vi "Make DLL Param(Read Storage Rsp).vi"(1 "Read Storage Rsp":T2) -> (0 "pRsp":T1)   [LabVIEW 8.6, in "Keyence LJ-V7000.lvlib"]
uses:
  Keyence LJ-V7000.lvlib
  Public/Clusters/Time.ctl
  Public/Clusters/Read Storage Rsp.ctl
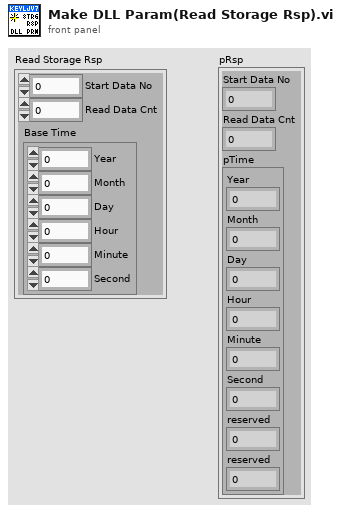
[diagram p1: front panel]
types:
  T1 = cluster{"Start Data No":u32, "Read Data Cnt":u32, "pTime":cluster{"Year":u8, "Month":u8, "Day":u8, "Hour":u8, "Minute":u8, "Second":u8, "reserved":u8, "reserved":u8}}
  T2 = typedef "Keyence LJ-V7000.lvlib/Read Storage Rsp.ctl" = cluster{"Start Data No":u32, "Read Data Cnt":u32, "Base Time":T3}
  T3 = typedef "Keyence LJ-V7000.lvlib/Time.ctl" = cluster{"Year":u8, "Month":u8, "Day":u8, "Hour":u8, "Minute":u8, "Second":u8}
  T4 = cluster{"Year":u8, "Month":u8, "Day":u8, "Hour":u8, "Minute":u8, "Second":u8, "reserved":u8, "reserved":u8}
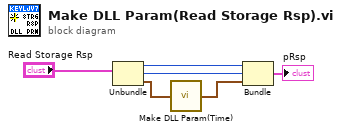
[diagram p0: block diagram]
diagram:
  n1 = Unbundle("Read Storage Rsp") -> ("Start Data No"=w4:u32, "Read Data Cnt"=w3:u32, "Base Time"=w5:T3)
  n2 = call "Make DLL Param(Time).vi"("Time"=w5) -> ("pTime"=w2:T4)
  n3 = Bundle("Start Data No"=w4, "Read Data Cnt"=w3, "pTime"=w2) -> (→"pRsp":T1)  [unwired: 1 in]
